vi "circular_roi_detect(SubVI).vi"(8 "error in (no error)":errorcluster, 11 "image in":T2) -> (0 "error out":errorcluster, 3 "ROI Descriptor":T1 {"Contours"."Type" items=["No Selection", "Point", "Line", "Rectangle", "Oval", "Polygon", "Freehand Region", "Annulus", "Unused2", "Unused3", "Broken Line", "Freehand Line", "Rotated Rectangle"]})   [LabVIEW 2020]
doc: "Cerca un cerchio all'interno dell'immagine e ne deduce una ROI circolare. Ha bisogno in ingresso di un cerchio pieno ben distinguibile dallo sfondo."
uses:
  <vilib>/vision/Image Controls.llb/IMAQ Image.ctl
  <vilib>/vision/NI_Vision_Development_Module.lvlib
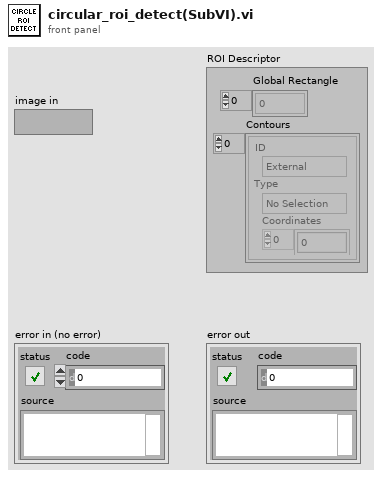
[diagram p1: front panel]
types:
  T1 = typedef "ROI Descriptor" = cluster{"Global Rectangle":i32[], "Contours":cluster{"ID":enum32{"External", "Internal"}, "Type":u32, "Coordinates":i32[]}[]}
  T2 = typedef "IMAQ Image.ctl" = refnum<image>
  T3 = typedef "IMAQ Circle" = cluster{"Center X":i32, "Center Y":i32, "Inner Radius":i32, "Outer Radius":i32, "Start Angle":dbl, "End Angle":dbl}
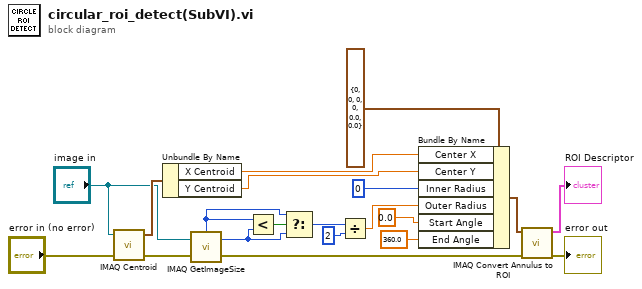
[diagram p0: block diagram]
diagram:
  n1 = call "IMAQ Centroid"("error in (no error)"="error in (no error)", "Image"="image in") -> ("error out"=w5:errorcluster, "Centroid"=w9:cluster{"X Centroid":sgl, "Y Centroid":sgl})  [unwired: 2 in]
  n2 = Unbundle By Name(w9) -> ("X Centroid"=w10:sgl, "Y Centroid"=w11:sgl)
  n3 = call "IMAQ GetImageSize"("Image"="image in", "error in (no error)"=w5) -> ("Y Resolution"=w2:i32, "X Resolution"=w3:i32, "error out"=w4:errorcluster)  [unwired: 2 in]
  n4 = Less?(x=w3, y=w2) -> (x < y?=w15:bool)
  n5 = Select(t=w3, s=w15, f=w2) -> (s? t:f=w16:i32)
  n6 = Divide(x=w16, y=2) -> (x/y=w18:dbl)
  n7 = Bundle By Name(cluster=T3 {"Center X"=0, "Center Y"=0, "Inner Radius"=0, "Outer Radius"=0, "Start Angle"=0.0, "End Angle"=0.0} ("Annulus"), "Center X"=w10, "Center Y"=w11, "Inner Radius"=0, "Outer Radius"=w18, "Start Angle"=0.0, "End Angle"=360.0) -> (w19:T3)
  n8 = call "IMAQ Convert Annulus to ROI"("error in (no error)"=w4, "Annulus"=w19) -> ("error out"=→"error out":errorcluster, "ROI Descriptor"=→"ROI Descriptor":T1)  [unwired: 7 in]
